vi "SQL_request.vi"   [LabVIEW 2020, in "DB.lvclass"]
uses:
  DB.lvclass
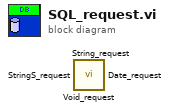
[diagram p0: block diagram]
diagram:
  n1 = call-dynamic "Void_request.vi"() -> ()  [unwired: 10 in, 2 out]
  n2 = call-dynamic "String_request.vi"() -> ()  [unwired: 9 in, 3 out]
  n3 = call-dynamic "StringS_request.vi"() -> ()  [unwired: 8 in, 4 out]
  n4 = call-dynamic "Date_request.vi"() -> ()  [unwired: 9 in, 3 out]
